vi "Update Packaging Instructions.vi"(8 "error in (no error)":errorcluster, 10 "Output Parameters":T2, 11 "Data Value Reference in":T1) -> (0 "error out":errorcluster, 2 "Packaging Instructions":string[](array[string]), 3 "Data Value Reference out":T1)   [LabVIEW 2023]
uses:
  <vilib>/Noffz/UTP IO/UTP IO Library/Typedefs/Session Handle.ctl
  <vilib>/Noffz/UTP IO/UTP IO Library/UTP IO Pool Session.lvclass
  <vilib>/Noffz/UTP IO/UTP IO Library/methods/poly/plc/Write PLC Variable (String).vi
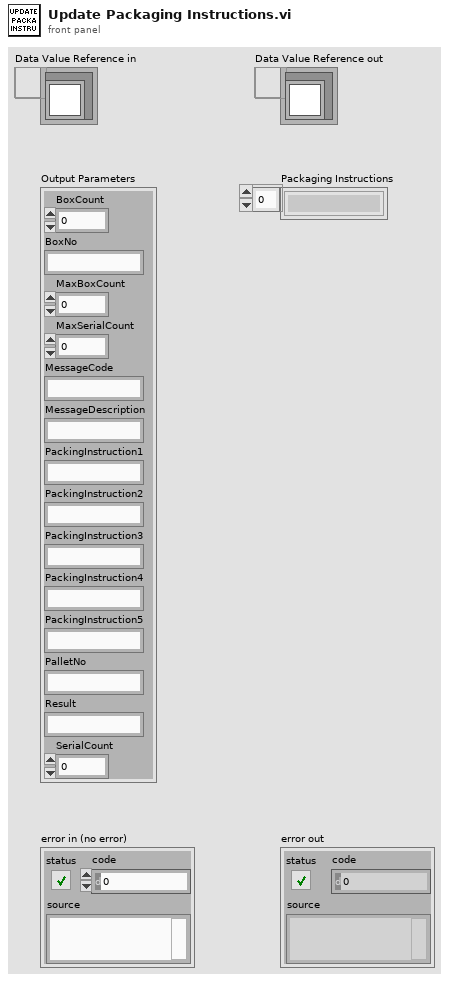
[diagram p1: front panel]
types:
  T1 = typedef "UTP IO Library.lvlib/UTP IO Pool Session.lvclass/Session Handle.ctl" = refnum<data-value>
  T2 = cluster{"BoxCount":i32, "BoxNo":string, "MaxBoxCount":i32, "MaxSerialCount":i32, "MessageCode":string, "MessageDescription":string, "PackingInstruction1":string, "PackingInstruction2":string, "PackingInstruction3":string, "PackingInstruction4":string, "PackingInstruction5":string, "PalletNo":string, "Result":string, "SerialCount":i32}
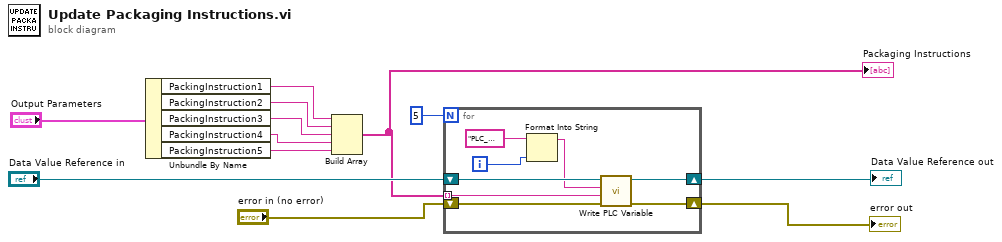
[diagram p0: block diagram]
diagram:
  n1 = Unbundle By Name("Output Parameters") -> ("PackingInstruction1"=w6:string, "PackingInstruction2"=w5:string, "PackingInstruction3"=w4:string, "PackingInstruction4"=w3:string, "PackingInstruction5"=w2:string)
  n2 = Build Array(w6, w5, w4, w3, w2) -> (w1:string[])
  "Packaging Instructions" <- w1
  n3 = for {
    N: 5 -> [_]
    shift-right: [w19] -> w9
    shift-left: "Data Value Reference in" -> [w20]
    shift-right: [w17] -> w11
    shift-left: "error in (no error)" -> [w18]
    tunnel: w1 -> [w13] mode=indexing
    i -> [w14]
    n4 = Format Into String(initial string="PLC_Packaging_Instruction_" ("variable name"), w14) -> (resulting string=w15:string)  [unwired: 2 in, 1 out]
    n5 = call-poly <vilib>:"Write PLC Variable.vi"("error in (no error)"=w18, "value"=w13, "variable name"=w15, "UTP IO Session in"=w20) -> ("error out"=w17:errorcluster, "UTP IO Session out"=w19:T1)  [unwired: 6 in]
  }
  "error out" <- w11
  "Data Value Reference out" <- w9
